vi "Eth Status Read statuses.vi"(8 "error in (no error)":errorcluster, 9 "Lenght (1)":i32=1, 10 "N (0)":i32, 11 "Status References":T1) -> (0 "error out":errorcluster, 1 "States":T2[](array[typedef]))   [LabVIEW 2019, in "Eth Status.lvlib"]
uses:
  Eth Status.lvlib
  MB_TCP2/MB_TCP_State.ctl
  Ctl/ICPCON Status.ctl
  MB_TCP2/MB_TCP.lvclass
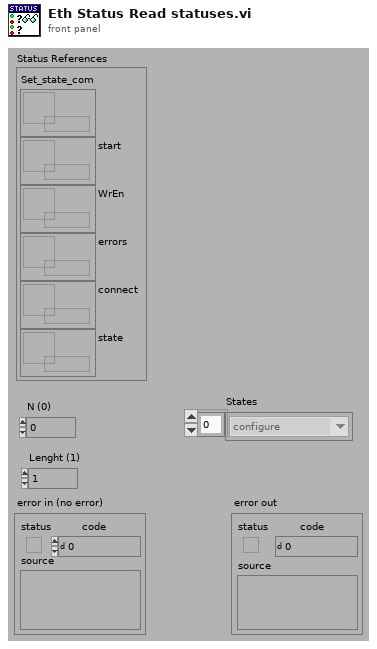
[diagram p1: front panel]
types:
  T1 = typedef "Eth Status.lvlib/ICPCON Status.ctl" = cluster{"Set_state_com":refnum<data-value>, "start":refnum<data-value>, "WrEn":refnum<data-value>, "errors":refnum<data-value>, "connect":refnum<data-value>, "state":refnum<data-value>}
  T2 = typedef "MB_TCP.lvclass/MB_TCP_State.ctl" = enum8{"initialization", "redefine", "standby", "connect", "wait to reconnect", "wait to reset timeout", "configure", "requests", "close connection", "stop"}
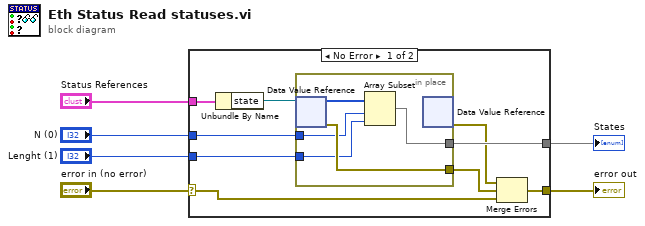
[diagram p0: block diagram]
diagram:
  n1 = case shown="No Error" "error in (no error)" {
    selector: "error in (no error)" -> [w7 w21]
    tunnel: [w12 w21] -> w1
    tunnel: [w15 _] -> w2
    tunnel: "N (0)" -> [w14 _]
    tunnel: "Status References" -> [w13 _]
    tunnel: "Lenght (1)" -> [w9 _]
    frame No Error {
      n2 = Unbundle By Name(w13) -> ("state"=w8:refnum<data-value>)
      n3 = in-place {
        in-place-border: w14 -> [w18]
        in-place-border: [w16] -> w15
        in-place-border: [w20] -> w10
        in-place-border: w9 -> [w17]
        n4 = in-place-dvr #1(w8) -> (w19:T2[], w20:errorcluster)
        n5 = Array Subset(array=w19, index=w18, length=w17) -> (w16:T2[])
        n6 = in-place-dvr #1() -> (w11:errorcluster)  [unwired: 1 in, 1 out]
      }
      n7 = Merge Errors(w11, w10, w7) -> (w12:errorcluster)
    }
    frame Error {
    }
  }
  "error out" <- w1
  "States" <- w2
